vi "Get_Box_NO_Loop.vi"(7 "Dark Blue \nFrame":T2={"Rmax"=14.0, "Rmin"=0.0, "Gmax"=42.0, "Gmin"=0.0, "Bmax"=126.0, "Bmin"=121.0}, 8 "Error in (no error)":errorcluster, 11 "Path to PNG file":path) -> (0 "Error out":errorcluster, 2 "BillardBox":T1)   [LabVIEW 2019]
doc: "Get_Box_NO_Loop.vi\nFind the coordinates of billard box by vectorisation (without loop).\nInput : -Path to PNG file\n -Dark Blue Frame containing the range of colors of the edge \n -Error in\nOutput : -BillardBox containing the coordinates of the billard box\n -Error out"
panel:
  in  "Initial BillardBox":T1
  # "127,93,748,408"
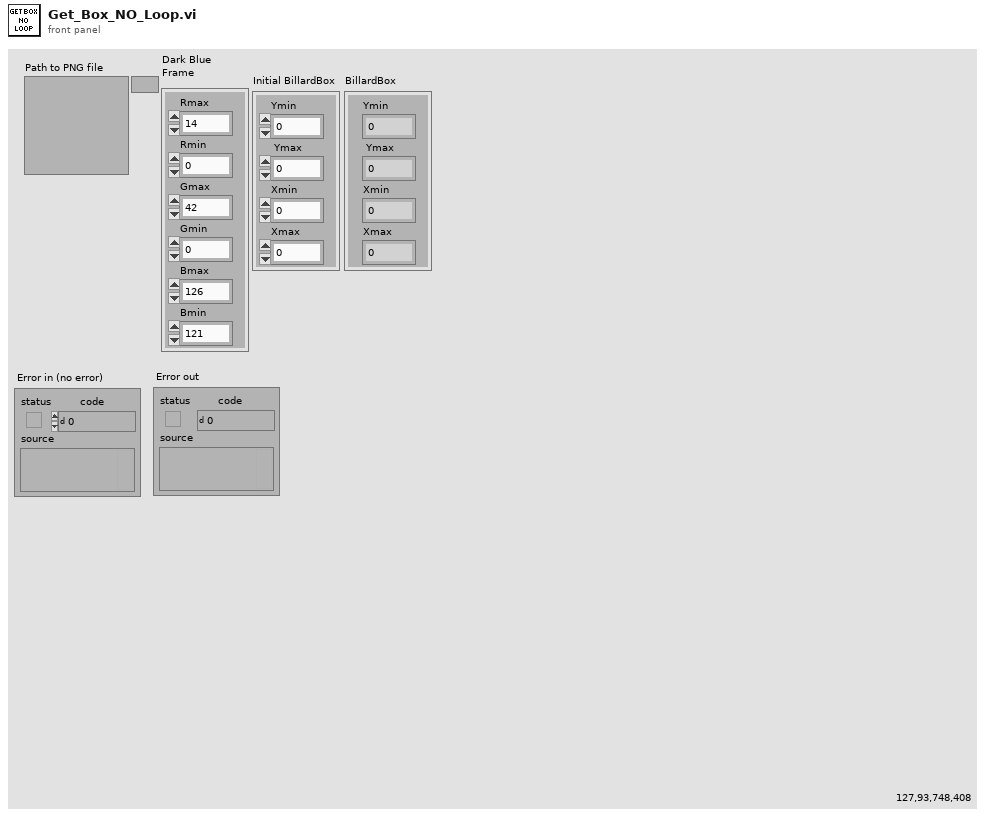
[diagram p1: front panel]
types:
  T1 = cluster{"Ymin":dbl, " Ymax":dbl, "Xmin":dbl, "Xmax":dbl}
  T2 = cluster{"Rmax":dbl, "Rmin":dbl, "Gmax":dbl, "Gmin":dbl, "Bmax":dbl, "Bmin":dbl}
  T3 = typedef "imagedata.ctl" = cluster{"image type":i32, "image depth":i32, "image":u8[], "mask":u8[], "colors":u32[], "Rectangle":cluster{"left":i16, "top":i16, "right":i16, "bottom":i16}}
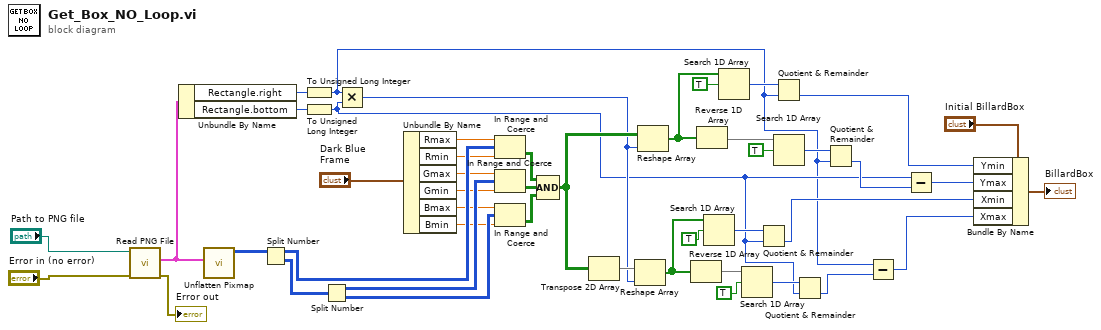
[diagram p0: block diagram]
diagram:
  n1 = call <vilib>:"Read PNG File.vi"("error in (no error)"="Error in (no error)", "path to PNG file"="Path to PNG file") -> ("error out"=→"Error out":errorcluster, "image data"=w46:T3)  [unwired: 7 in, 1 out]
  n2 = Unbundle By Name(w46) -> ("Rectangle.right"=w45:i16, "Rectangle.bottom"=w44:i16)
  n3 = call <vilib>:"Unflatten Pixmap.vi"("image data"=w46) -> ("24-bit pixmap"=w31:u32[][])  [unwired: 4 in, 6 out]
  n4 = Split Number(x=w31) -> (hi(x)=w39:u16[][], lo(x)=w43:u16[][])
  n5 = To Unsigned Long Integer(number=w45) -> (unsigned 32bit integer=w1:u32)
  n6 = To Unsigned Long Integer(number=w44) -> (unsigned 32bit integer=w2:u32)
  n7 = Split Number(x=w43) -> (hi(x)=w38:u8[][], lo(x)=w37:u8[][])
  n8 = Multiply(x=w1, y=w2) -> (x*y=w4:u32)
  n9 = Unbundle By Name("Dark Blue \nFrame") -> ("Rmax"=w24:dbl, "Rmin"=w23:dbl, "Gmax"=w22:dbl, "Gmin"=w21:dbl, "Bmax"=w20:dbl, "Bmin"=w19:dbl)
  n10 = In Range and Coerce(upper limit=w24, x=w39, lower limit=w23) -> (In Range?=w42:bool[][])  [unwired: 1 out]
  n11 = In Range and Coerce(upper limit=w22, x=w38, lower limit=w21) -> (In Range?=w41:bool[][])  [unwired: 1 out]
  n12 = In Range and Coerce(upper limit=w20, x=w37, lower limit=w19) -> (In Range?=w40:bool[][])  [unwired: 1 out]
  n13 = Compound Arithmetic op=AND(w42, w41, w40) -> (w30:bool[][])
  n14 = Transpose 2D Array(2D array=w30) -> (transposed array=w29:bool[][])
  n15 = Reshape Array(w29, w4) -> (w16:bool[])
  n16 = Reshape Array(w30, w4) -> (w18:bool[])
  n17 = Reverse 1D Array(array=w16) -> (reversed array=w13:bool[])
  n18 = Reverse 1D Array(array=w18) -> (reversed array=w17:bool[])
  n19 = Search 1D Array(1D array=w16, element=TRUE) -> (index of element=w32:i32)  [unwired: 1 in]
  n20 = Search 1D Array(1D array=w18, element=TRUE) -> (index of element=w35:i32)  [unwired: 1 in]
  n21 = Search 1D Array(1D array=w13, element=TRUE) -> (index of element=w15:i32)  [unwired: 1 in]
  n22 = Quotient & Remainder(x=w32, y=w2) -> (floor(x/y)=w7:u32)  [unwired: 1 out]
  n23 = Quotient & Remainder(x=w35, y=w1) -> (floor(x/y)=w10:u32)  [unwired: 1 out]
  n24 = Search 1D Array(1D array=w17, element=TRUE) -> (index of element=w5:i32)  [unwired: 1 in]
  n25 = Quotient & Remainder(x=w15, y=w2) -> (floor(x/y)=w14:u32)  [unwired: 1 out]
  n26 = Quotient & Remainder(x=w5, y=w1) -> (floor(x/y)=w6:u32)  [unwired: 1 out]
  n27 = Subtract(x=w1, y=w14) -> (x-y=w8:u32)
  n28 = Subtract(x=w2, y=w6) -> (x-y=w9:u32)
  n29 = Bundle By Name(cluster="Initial BillardBox", "Ymin"=w10, "Ymax"=w9, "Xmin"=w7, "Xmax"=w8) -> (→"BillardBox":T1)
